vi "prometheus.vi"   [LabVIEW 2014, in "Janga.lvrbt"]
uses:
  Janga.lvrbt
  <vilib>/NXT/Block Support/NXT_OutputPort.ctl
  <vilib>/NXT/NXTIO Xnodes/NXTIONodeSubVIs/NXTMotorRunDistance.vi
  <vilib>/NXT/Subs/LVHSConnector.ctl
  <vilib>/NXT/NXTIO Xnodes/AddressXNode/NXTIOAddress.xnode
  <vilib>/NXT/NXTIO Xnodes/NXTIOXNode/NXTIO.xnode
  <vilib>/NXT/LegoClasses/BrickReference/BrickReference.lvclass
types:
  T1 = typedef "NXT_OutputPort.ctl" = u8
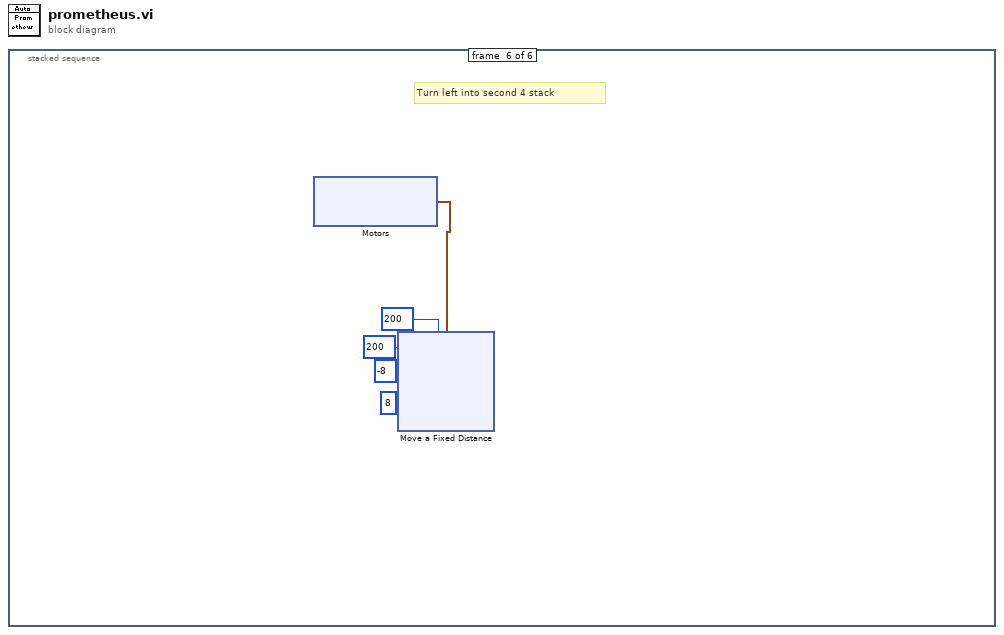
[diagram p0: block diagram]
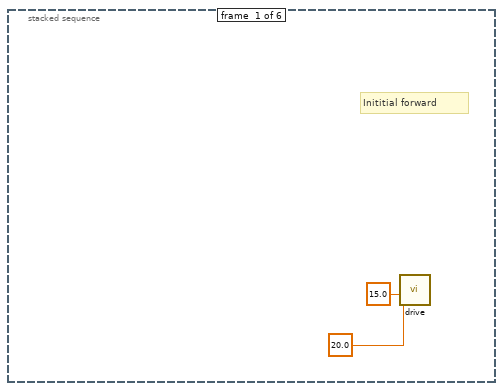
[diagram p2: hidden frame]
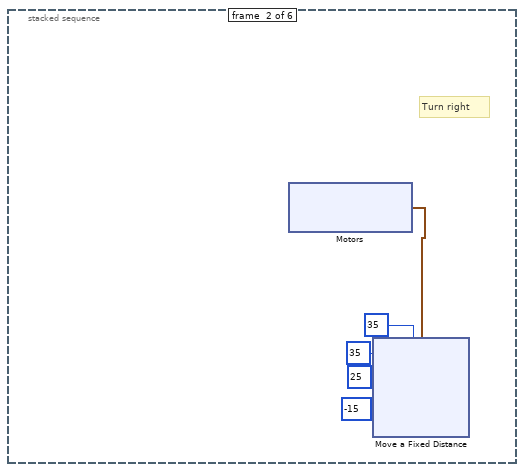
[diagram p3: hidden frame]
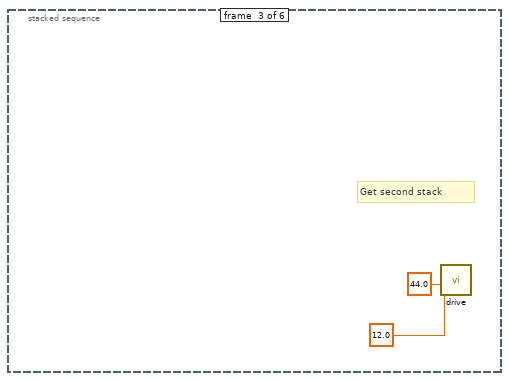
[diagram p4: hidden frame]
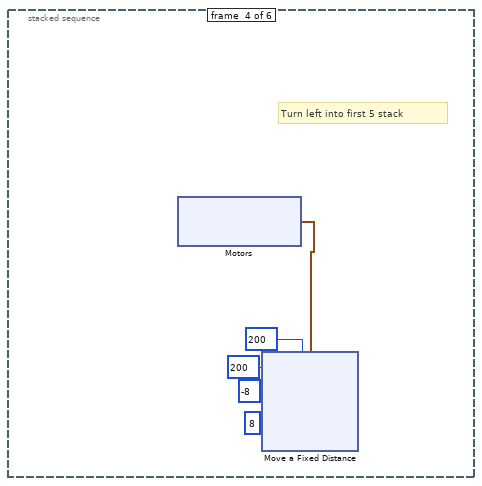
[diagram p5: hidden frame]
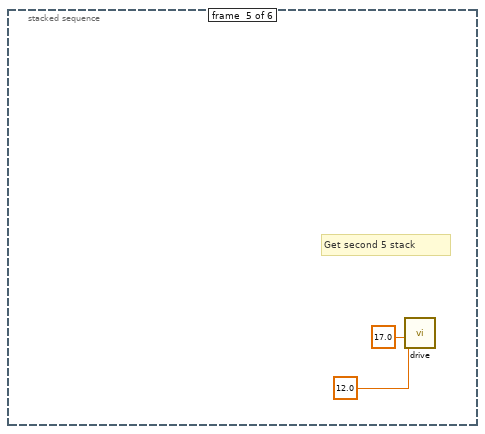
[diagram p6: hidden frame]
diagram:
  n1 = stacked-sequence {
    frame #0 {
      # "Inititial forward"
      n2 = call "drive.vi"("Speed"=20.0, "Distance (cm)"=15.0) -> ()  [unwired: 10 in]
    }
    frame #1 {
      # "Turn right"
      n3 = xnode "Motors"() -> ("Motor"=w7:cluster{"Port":T1, "Port":T1})
      n4 = xnode "Move a Fixed Distance"("Speed 2"=i8 -15, "Speed 1"=i8 25, "Distance 2"=35, "Distance 1"=35, "Motors"=w7) -> ()  [unwired: 1 in, 1 out]
    }
    frame #2 {
      # "Get second stack"
      n5 = call "drive.vi"("Speed"=12.0, "Distance (cm)"=44.0) -> ()  [unwired: 10 in]
    }
    frame #3 {
      # "Turn left into first 5 stack"
      n6 = xnode "Motors"() -> ("Motor"=w27:cluster{"Port":T1, "Port":T1})
      n7 = xnode "Move a Fixed Distance"("Speed 2"=i8 8, "Speed 1"=i8 -8, "Distance 2"=200, "Distance 1"=200, "Motors"=w27) -> ()  [unwired: 1 in, 1 out]
    }
    frame #4 {
      # "Get second 5 stack"
      n8 = call "drive.vi"("Speed"=12.0, "Distance (cm)"=17.0) -> ()  [unwired: 10 in]
    }
    frame #5 {
      # "Turn left into second 4 stack"
      n9 = xnode "Motors"() -> ("Motor"=w47:cluster{"Port":T1, "Port":T1})
      n10 = xnode "Move a Fixed Distance"("Speed 2"=i8 8, "Speed 1"=i8 -8, "Distance 2"=200, "Distance 1"=200, "Motors"=w47) -> ()  [unwired: 1 in, 1 out]
    }
  }
